vi "setup.vi"() -> ()   [LabVIEW 2010]
uses:
  <vilib>/Utility/config.llb/NI_LVConfig.lvlib
panel:
  out "Array":path[](array[path])
  out "WorkingDirectory":string
  out "autoexec":string
  in  "Soft":path caption="Программный WatchDog"
  in  "WDTpath":path caption="Аппаратный WatchDog"
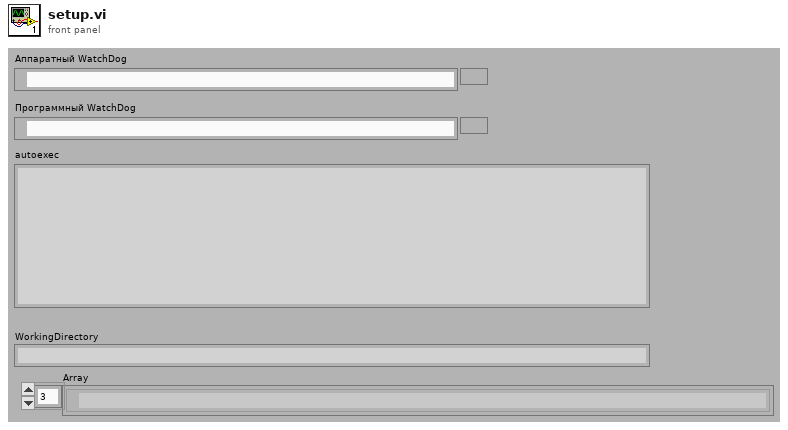
[diagram p1: front panel]
types:
  T1 = typedef "NI_LVConfig.lvlib/Config Data RefNum.ctl" = refnum<k1>
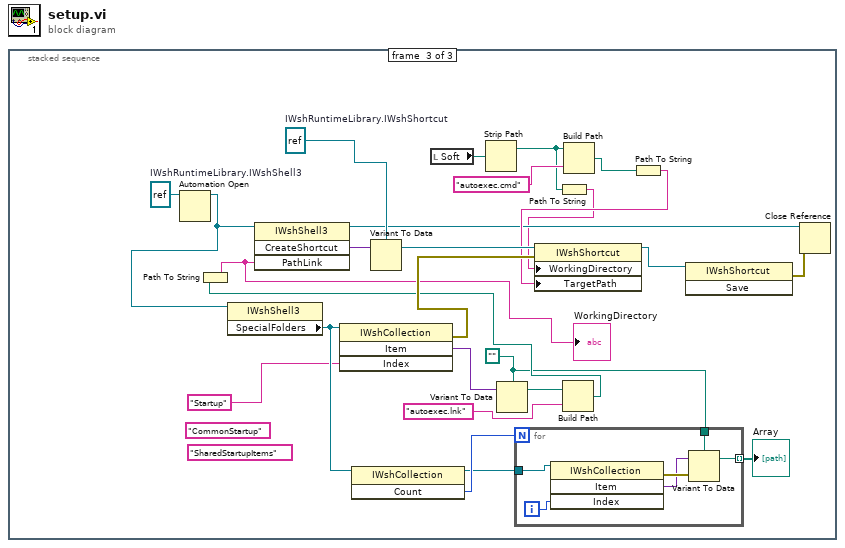
[diagram p0: block diagram]
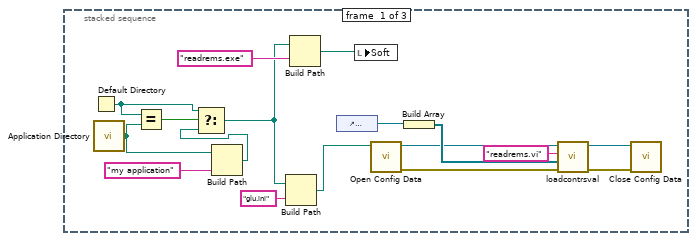
[diagram p2: hidden frame]
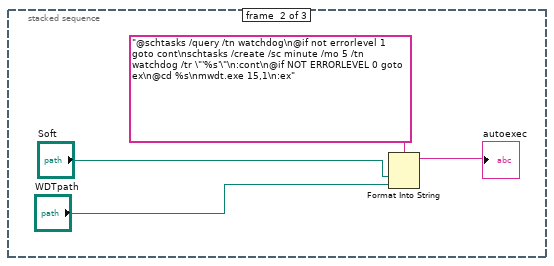
[diagram p3: hidden frame]
diagram:
  n1 = stacked-sequence {
    frame #0 {
      n2 = Default Directory() -> (w2:path)
      n3 = call <vilib>:"Application Directory.vi"() -> ("Application Directory"=w12:path)
      n4 = Equal?(x=w2, y=w12) -> (x = y?=w1:bool)
      n5 = Build Path(base path=w12, name or relative path="my application") -> (appended path=w14:path)
      n6 = Select(t=w2, s=w1, f=w14) -> (s? t:f=w15:path)
      n7 = Build Path(base path=w15, name or relative path="glu.ini") -> (appended path=w4:path)
      n8 = Build Path(base path=w15, name or relative path="readrems.exe" ("Section")) -> (appended path=w17:path)
      n9 = control-ref of="WDTpath"() -> (w6:refnum<vi>)
      n10 = local write "Soft"(w17) -> ()
      n11 = call <vilib>:"Open Config Data.vi"("configuration file path"=w4) -> ("error out"=w9:errorcluster, "refnum"=w5:T1)  [unwired: 8 in, 1 out]
      n12 = Build Array(w6) -> (w7:refnum<vi>[])
      n13 = call "loadcontrsval.vi"("error in"=w9, "Array"=w7, "Section"="readrems.vi", "refnum in"=w5) -> ("error out"=w10:errorcluster, "refnum out"=w11:T1)  [unwired: 1 in, 1 out]
      n14 = call <vilib>:"Close Config Data.vi"("error in (no error)"=w10, "refnum"=w11) -> ()  [unwired: 8 in, 2 out]
    }
    frame #1 {
      n15 = Format Into String(format string="@schtasks /query /tn watchdog\n@if not errorlevel 1 goto cont\nschtasks /create /sc minute /mo 5 /tn watchdog /tr \"'%s'\"\n:cont\n@if NOT ERRORLEVEL 0 goto ex\n@cd %s\nmwdt.exe 15,1\n:ex", "Soft", "WDTpath") -> (resulting string=→"autoexec":string)  [unwired: 2 in, 1 out]
    }
    frame #2 {
      (unwired) "SharedStartupItems"
      (unwired) "CommonStartup"
      w34 = path ""
      w45 = refnum<k7> refnum  # IWshRuntimeLibrary.IWshShortcut
      w47 = refnum<k7> refnum  # IWshRuntimeLibrary.IWshShell3
      n16 = Automation Open(Automation Refnum=w47) -> (Automation Refnum=w43:refnum<k7>)  [unwired: 3 in, 1 out]
      n17 = property class="IWshShell3"(reference=w43) -> ("SpecialFolders"=w37:refnum<k7>)  [unwired: 1 in, 2 out]
      n18 = invoke class="IWshCollection" method="Item"(reference=w37, "Index"="Startup") -> (error out=w42:errorcluster, "Item"=w41:variant)  [unwired: 2 in, 2 out]
      n19 = invoke class="IWshCollection" method="Count"(reference=w37) -> (reference out=w35:refnum<k7>, "Count"=w36:i32)  [unwired: 2 in, 1 out]
      n20 = local read "Soft"() -> (w30:path)
      n21 = Strip Path(path=w30) -> (stripped path=w23:path)  [unwired: 1 out]
      n22 = Variant To Data(Variant=w41, type=w34) -> (data=w40:path)  [unwired: 1 in, 1 out]
      n23 = for {
        N: w36 -> [_]
        tunnel: w35 -> [w53]
        tunnel: w34 -> [w49]
        tunnel: [w48] -> w33 mode=indexing
        i -> [w52]
        n24 = invoke class="IWshCollection" method="Item"(reference=w53, "Index"=w52) -> (error out=w51:errorcluster, "Item"=w50:variant)  [unwired: 2 in, 2 out]
        n25 = Variant To Data(error in=w51, Variant=w50, type=w49) -> (data=w48:path)  [unwired: 1 out]
      }
      "Array" <- w33
      n26 = Path To String(path=w23) -> (string=w22:string)
      n27 = Build Path(base path=w40, name or relative path="autoexec.lnk" ("PathLink")) -> (appended path=w38:path)
      n28 = Path To String(path=w38) -> (string=w32:string)
      "WorkingDirectory" <- w32
      n29 = invoke class="IWshShell3" method="CreateShortcut"(reference=w43, "PathLink"=w32) -> (reference out=w26:refnum<k7>, "CreateShortcut"=w46:variant)  [unwired: 2 in, 2 out]
      n30 = Variant To Data(Variant=w46, type=w45) -> (data=w44:refnum<k7>)  [unwired: 1 in, 1 out]
      n31 = Build Path(base path=w23, name or relative path="autoexec.cmd") -> (appended path=w28:path)
      n32 = Path To String(path=w28) -> (string=w27:string)
      n33 = property class="IWshShortcut"(reference=w44, error in=w42, "WorkingDirectory"=w22, "TargetPath"=w27) -> (reference out=w25:refnum<k7>)  [unwired: 1 out]
      n34 = invoke class="IWshShortcut" method="Save"(reference=w25) -> (error out=w24:errorcluster)  [unwired: 2 in, 2 out]
      n35 = Close Reference(reference=w26, error in (no error)=w24) -> ()  [unwired: 1 out]
    }
  }
